vi "Demodulacja_DSBFC_2.vi"(10 "Parametry_sygnalu_nosnego":T1, 11 "Sygnal_zmodulowany":dbl[](array[numeric])) -> (3 "Sygnal_zdemodulowany":dbl[](array[numeric]))   [LabVIEW 2020]
doc: "VI demoduluje sygnal zmodulowany metoda DSBFC wykorzystujac detekcje obwiedniowa wykorzystujaca transformate Hilberta"
uses:
  Kontrolki/Parametry_cosinusa.ctl
  <vilib>/Analysis/NI_AALPro.lvlib
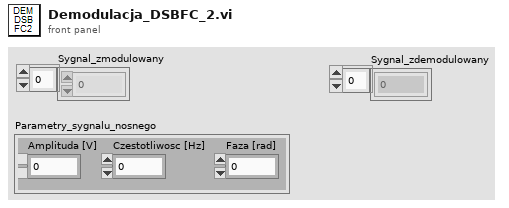
[diagram p1: front panel]
types:
  T1 = typedef "Parametry_cosinusa.ctl" = cluster{"Amplituda [V]":dbl, "Czestotliwosc [Hz] ":dbl, "Faza [rad]":dbl}
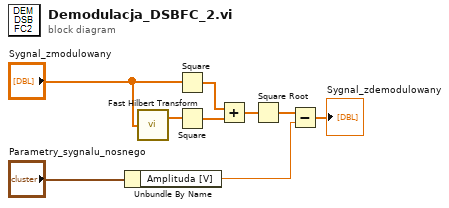
[diagram p0: block diagram]
diagram:
  n1 = Unbundle By Name("Parametry_sygnalu_nosnego") -> ("Amplituda [V]"=w2:dbl)
  n2 = call <vilib>:"Fast Hilbert Transform.vi"("X"="Sygnal_zmodulowany") -> ("Hilbert{X}"=w5:dbl[])  [unwired: 1 out]
  n3 = Square(x="Sygnal_zmodulowany") -> (x^2=w6:dbl[])
  n4 = Square(x=w5) -> (x^2=w7:dbl[])
  n5 = Add(x=w6, y=w7) -> (x+y=w9:dbl[])
  n6 = Square Root(x=w9) -> (sqrt(x)=w8:dbl[])
  n7 = Subtract(x=w8, y=w2) -> (x-y=→"Sygnal_zdemodulowany":dbl[])
